vi "CRYTime Array Interp Outside Range.vi"(8 "Decimating factor":i32, 9 "Sampling rate":dbl format="%.2f", 10 "Search range (ms)":string[](array[string]), 11 "Points in time":dbl[](array[numeric]) format="%.2f") -> (3 "Processed points in time":dbl[](array[numeric]) format="%.2f")   [LabVIEW 2013]
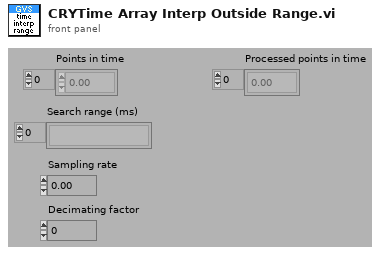
[diagram p1: front panel]
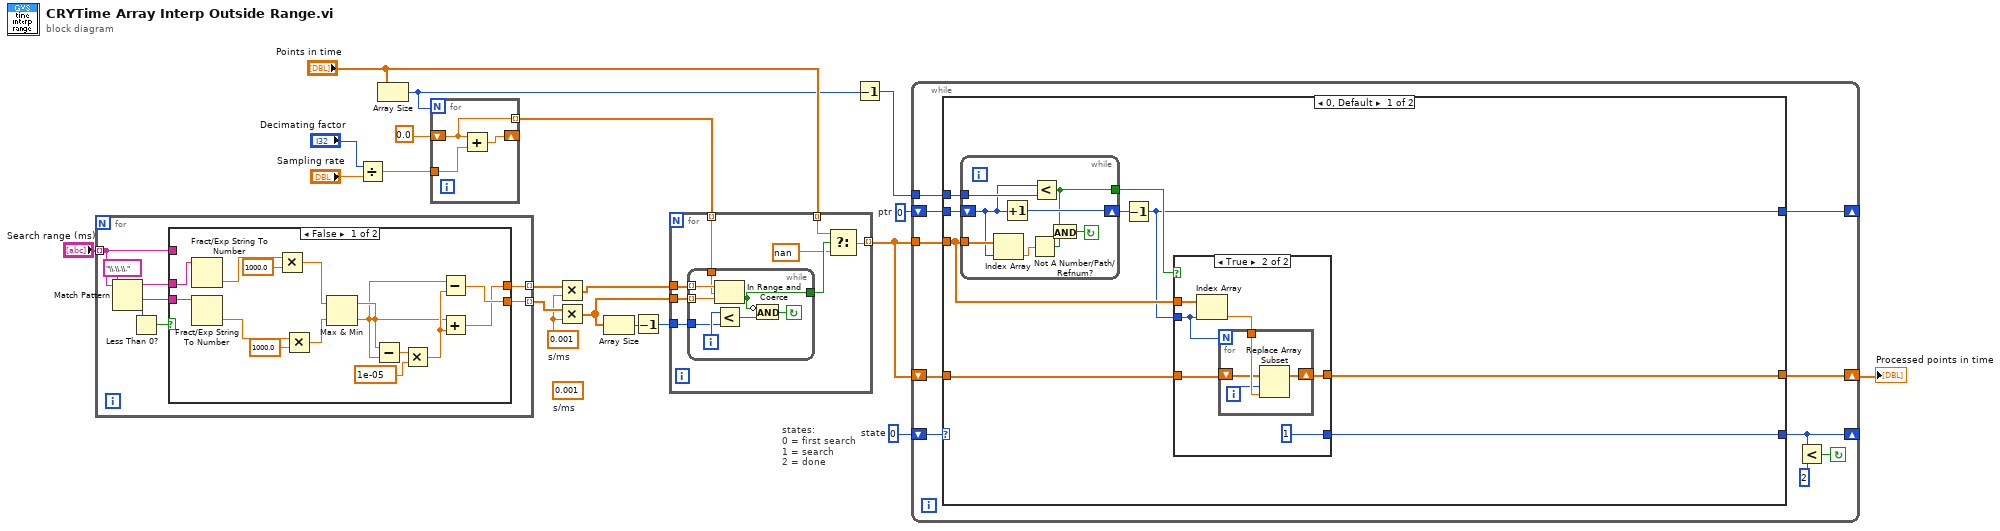
[diagram p0: block diagram]
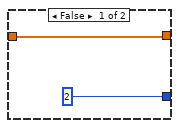
[diagram p2: hidden frame]
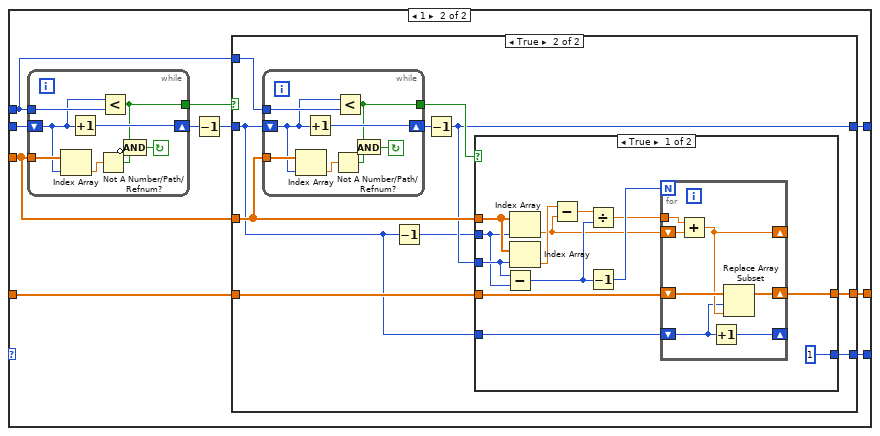
[diagram p3: hidden frame]
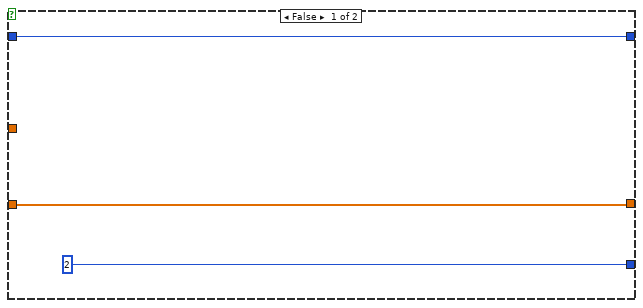
[diagram p4: hidden frame]
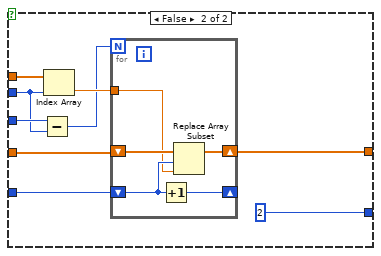
[diagram p5: hidden frame]
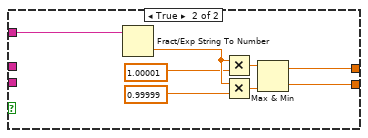
[diagram p6: hidden frame]
diagram:
  (unwired) 0.001  # s/ms
  w7 = 0  # ptr
  w8 = 0  # state
  w14 = 0.001  # s/ms
  # "states:\n0 = first search\n1 = search\n2 = done"
  n1 = for {
    tunnel: "Search range (ms)" -> [w23] mode=indexing
    tunnel: [w22] -> w16 mode=indexing
    tunnel: [w21] -> w15 mode=indexing
    n2 = Match Pattern(string=w23, regular expression="\\.\\.\\.") -> (before substring=w24:string, after substring=w25:string, offset past match=w27:i32)  [unwired: 2 out]
    n3 = Less Than 0?(x=w27) -> (x < 0?=w26:bool)
    n4 = case shown="False" w26 {
      tunnel: w25 -> [w43 _]
      tunnel: w24 -> [w42 _]
      tunnel: w23 -> [_ w51]
      tunnel: [w38 w45] -> w22
      tunnel: [w39 w44] -> w21
      frame False {
        n5 = Fract/Exp String To Number(string=w42) -> (number=w34:dbl)  [unwired: 4 out]
        n6 = Fract/Exp String To Number(string=w43) -> (number=w31:dbl)  [unwired: 4 out]
        n7 = Multiply(x=w34, y=1000.0) -> (x*y=w29:dbl)
        n8 = Multiply(x=w31, y=1000.0) -> (x*y=w30:dbl)
        n9 = Max & Min(x=w29, y=w30) -> (max(x,y)=w37:dbl, min(x,y)=w36:dbl)
        n10 = Subtract(x=w37, y=w36) -> (x-y=w41:dbl)
        n11 = Multiply(x=w41, y=1e-05) -> (x*y=w40:dbl)
        n12 = Subtract(x=w36, y=w40) -> (x-y=w39:dbl)
        n13 = Add(x=w37, y=w40) -> (x+y=w38:dbl)
      }
      frame True {
        n14 = Fract/Exp String To Number(string=w51) -> (number=w50:dbl)  [unwired: 4 out]
        n15 = Multiply(x=w50, y=1.00001) -> (x*y=w47:dbl)
        n16 = Multiply(x=w50, y=0.99999) -> (x*y=w46:dbl)
        n17 = Max & Min(x=w47, y=w46) -> (max(x,y)=w45:dbl, min(x,y)=w44:dbl)
      }
    }
  }
  n18 = Divide(x="Decimating factor", y="Sampling rate") -> (x/y=w1:dbl)
  n19 = Array Size(array="Points in time") -> (size(s)=w6:i32)
  n20 = for {
    N: w6 -> [_]
    shift-right: [w53] -> _
    shift-left: 0.0 -> [w52]
    tunnel: w1 -> [w54]
    tunnel: [w52] -> w11 mode=indexing
    n21 = Add(x=w52, y=w54) -> (x+y=w53:dbl)
  }
  n22 = Multiply(x=w16, y=w14) -> (x*y=w13:dbl[])
  n23 = Multiply(x=w15, y=w14) -> (x*y=w12:dbl[])
  n24 = Array Size(array=w12) -> (size(s)=w20:i32)
  n25 = Decrement(x=w20) -> (x-1=w19:i32)
  n26 = for {
    tunnel: w13 -> [w62]
    tunnel: w12 -> [w61]
    tunnel: w19 -> [w60]
    tunnel: w11 -> [w59] mode=indexing
    tunnel: "Points in time" -> [w57] mode=indexing
    tunnel: [w55] -> w9 mode=indexing
    n27 = while {
      tunnel: w62 -> [w70] mode=indexing
      tunnel: w61 -> [w69] mode=indexing
      tunnel: w60 -> [w67]
      tunnel: [w64] -> w58
      tunnel: w59 -> [w63]
      i -> [w68]
      stop <- w65 continue-if-true
      n28 = In Range and Coerce(upper limit=w70, x=w63, lower limit=w69) -> (In Range?=w64:bool)  [unwired: 1 out]
      n29 = Less?(x=w68, y=w67) -> (x < y?=w66:bool)
      n30 = Compound Arithmetic op=AND(invert w64, w66) -> (w65:bool)
    }
    n31 = Select(t=w57, s=w58, f=nan) -> (s? t:f=w55:dbl)
  }
  n32 = Decrement(x=w6) -> (x-1=w5:i32)
  n33 = while {
    tunnel: w9 -> [w79]
    shift-right: [w74] -> w4
    shift-left: w9 -> [w75]
    shift-right: [w73] -> _
    shift-left: w8 -> [w80]
    shift-right: [w76] -> _
    shift-left: w7 -> [w77]
    tunnel: w5 -> [w78]
    stop <- w71 continue-if-true
    n34 = case shown="0, Default" w80 {
      tunnel: w79 -> [w83 w114]
      tunnel: w78 -> [w89 w111]
      tunnel: w77 -> [w88 w119]
      tunnel: [w82 w110] -> w76
      tunnel: [w86 w117] -> w73
      tunnel: w75 -> [w84 w115]
      tunnel: [w81 w112] -> w74
      frame 0, Default {
        n35 = while {
          tunnel: w83 -> [w109]
          tunnel: w89 -> [w107]
          shift-right: [w105] -> w87
          shift-left: w88 -> [w102]
          tunnel: [w103] -> w85
          stop <- w106 continue-if-true
          n36 = Index Array(array=w109, index=w102) -> (element=w108:dbl)
          n37 = Increment(x=w102) -> (x+1=w105:i32)
          n38 = Not A Number/Path/Refnum?(number/path/refnum=w108) -> (NaN/Path/Refnum?=w104:bool)
          n39 = Less?(x=w102, y=w107) -> (x < y?=w103:bool)
          n40 = And(x=w103, y=w104) -> (x .and. y?=w106:bool)
        }
        n41 = Decrement(x=w87) -> (x-1=w82:i32)
        n42 = case shown="True" w85 {
          tunnel: [2 1] -> w86
          tunnel: w84 -> [w90 w94]
          tunnel: w83 -> [_ w96]
          tunnel: w82 -> [_ w95]
          tunnel: [w90 w92] -> w81
          frame False {
          }
          frame True {
            n43 = Index Array(array=w96, index=w95) -> (element=w93:dbl)
            n44 = for {
              N: w95 -> [_]
              shift-right: [w99] -> w92
              shift-left: w94 -> [w100]
              tunnel: w93 -> [w101]
              i -> [w98]
              n45 = Replace Array Subset(array=w100, new element=w101, index=w98) -> (w99:dbl[])
            }
          }
        }
      }
      frame 1 {
        n46 = while {
          tunnel: w114 -> [w182]
          tunnel: w111 -> [w180]
          shift-right: [w179] -> w118
          shift-left: w119 -> [w175]
          tunnel: [w177] -> w116
          stop <- w176 continue-if-true
          n47 = Index Array(array=w182, index=w175) -> (element=w181:dbl)
          n48 = Increment(x=w175) -> (x+1=w179:i32)
          n49 = Not A Number/Path/Refnum?(number/path/refnum=w181) -> (NaN/Path/Refnum?=w178:bool)
          n50 = Less?(x=w175, y=w180) -> (x < y?=w177:bool)
          n51 = Compound Arithmetic op=AND(w177, invert w178) -> (w176:bool)
        }
        n52 = Decrement(x=w118) -> (x-1=w113:i32)
        n53 = case shown="True" w116 {
          tunnel: [2 w123] -> w117
          tunnel: w115 -> [w121 w129]
          tunnel: w114 -> [_ w128]
          tunnel: w113 -> [w120 w124]
          tunnel: [w121 w125] -> w112
          tunnel: w111 -> [_ w132]
          tunnel: [w120 w127] -> w110
          frame False {
          }
          frame True {
            n54 = while {
              tunnel: w128 -> [w174]
              tunnel: w132 -> [w172]
              shift-right: [w170] -> w131
              shift-left: w124 -> [w167]
              tunnel: [w168] -> w130
              stop <- w171 continue-if-true
              n55 = Index Array(array=w174, index=w167) -> (element=w173:dbl)
              n56 = Increment(x=w167) -> (x+1=w170:i32)
              n57 = Not A Number/Path/Refnum?(number/path/refnum=w173) -> (NaN/Path/Refnum?=w169:bool)
              n58 = Less?(x=w167, y=w172) -> (x < y?=w168:bool)
              n59 = And(x=w168, y=w169) -> (x .and. y?=w171:bool)
            }
            n60 = Decrement(x=w124) -> (x-1=w126:i32)
            n61 = Decrement(x=w131) -> (x-1=w127:i32)
            n62 = case shown="True" w130 {
              tunnel: w129 -> [w135 w153]
              tunnel: w128 -> [w145 w161]
              tunnel: w126 -> [w141 w155]
              tunnel: w127 -> [w142 w156]
              tunnel: [w133 w160] -> w125
              tunnel: w124 -> [w137 w159]
              tunnel: [1 2] -> w123
              frame True {
                n63 = Subtract(x=w142, y=w141) -> (x-y=w140:i32)
                n64 = Index Array(array=w145, index=w141) -> (element=w134:dbl)
                n65 = Index Array(array=w145, index=w142) -> (element=w144:dbl)
                n66 = Subtract(x=w144, y=w134) -> (x-y=w143:dbl)
                n67 = Divide(x=w143, y=w140) -> (x/y=w138:dbl)
                n68 = Decrement(x=w140) -> (x-1=w139:i32)
                n69 = for {
                  N: w139 -> [_]
                  shift-right: [w151] -> w133
                  shift-left: w135 -> [w152]
                  shift-right: [w148] -> _
                  shift-left: w134 -> [w150]
                  tunnel: w138 -> [w149]
                  shift-right: [w146] -> _
                  shift-left: w137 -> [w147]
                  n70 = Add(x=w149, y=w150) -> (x+y=w148:dbl)
                  n71 = Increment(x=w147) -> (x+1=w146:i32)
                  n72 = Replace Array Subset(array=w152, new element=w148, index=w147) -> (w151:dbl[])
                }
              }
              frame False {
                n73 = Subtract(x=w156, y=w155) -> (x-y=w154:i32)
                n74 = Index Array(array=w161, index=w155) -> (element=w157:dbl)
                n75 = for {
                  N: w154 -> [_]
                  shift-right: [w165] -> w160
                  shift-left: w153 -> [w166]
                  shift-right: [w163] -> _
                  shift-left: w159 -> [w164]
                  tunnel: w157 -> [w162]
                  n76 = Increment(x=w164) -> (x+1=w163:i32)
                  n77 = Replace Array Subset(array=w166, new element=w162, index=w164) -> (w165:dbl[])
                }
              }
            }
          }
        }
      }
    }
    n78 = Less?(x=w73, y=2) -> (x < y?=w71:bool)
  }
  "Processed points in time" <- w4
